vi "Image Indicator Ref.vi"(8 "error in (no error)":errorcluster, 10 "Image Refnum":refnum<vi>, 11 "Controller in":refnum<class "Controller.lvclass">) -> (0 "error out":errorcluster, 3 "Controller out":refnum<class "Controller.lvclass">)   [LabVIEW 2022 SP3, in "Controller.lvlib" / "Controller.lvclass"]
uses:
  Controller.lvclass
  Controller.lvclass/Controller.ctl
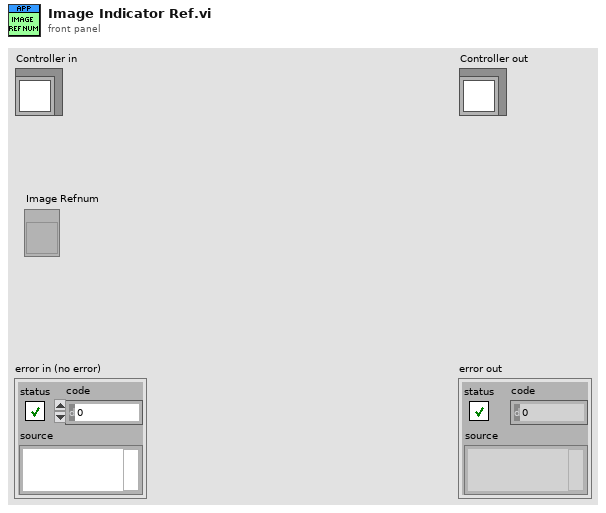
[diagram p1: front panel]
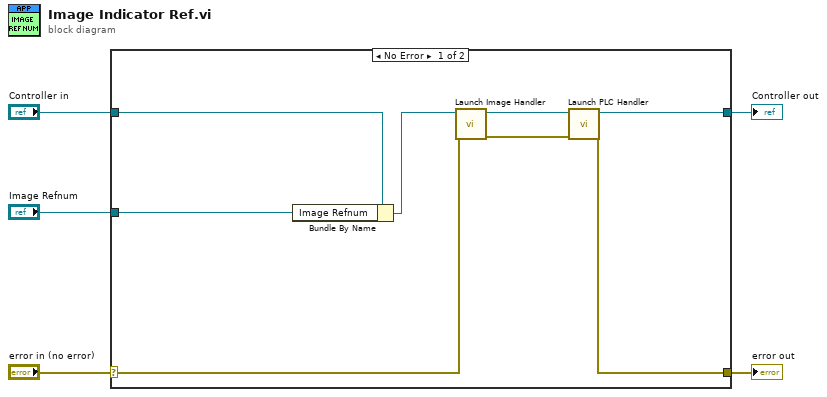
[diagram p0: block diagram]
diagram:
  n1 = case shown="No Error" "error in (no error)" {
    selector: "error in (no error)" -> [w8 w15]
    tunnel: [w6 w15] -> w4
    tunnel: [w9 w14] -> w2
    tunnel: "Controller in" -> [w13 w14]
    tunnel: "Image Refnum" -> [w11 _]
    frame No Error {
      n2 = Bundle By Name(cluster=w13, "Image Refnum"=w11) -> (w12:refnum<class "Controller.lvclass">)
      n3 = call "Launch Image Handler.vi"("error in (no error)"=w8, "Controller in"=w12) -> ("error out"=w7:errorcluster, "Controller out"=w10:refnum<class "Controller.lvclass">)  [unwired: 8 in]
      n4 = call "Launch PLC Handler.vi"("error in (no error)"=w7, "Controller in"=w10) -> ("error out"=w6:errorcluster, "Controller out"=w9:refnum<class "Controller.lvclass">)  [unwired: 8 in]
    }
    frame Error {
    }
  }
  "error out" <- w4
  "Controller out" <- w2
